vi "VeerAnemometers.vi"() -> ()   [LabVIEW 2011]
doc: "Use this VI with the UDP Sender VI. Run this VI first.\n\nThe UDP protocol differs from TCP in that there is no error-checking with the packets of information that are sent, and thus no guarantee whatsoever that an intended recipient will actually receive a given piece of data.\n\nUDP does offer the ability to \"broadcast\" data across a network--simply specify an IP Address of all ones (255.255.255.255) to attempt to broadcast information network-wide. Keep in mind that routers and other network hardware will generally refuse to forward the broadcast beyond certain points, so the extent of the broadcast will in practice be limited."
panel:
  out "Windspeed m/s 2":dbl(slide) scale=0.0..20.0
  out "Windspeed m/s":dbl(slide) scale=0.0..20.0
  out "Wind Direction":cluster{dbl, dbl}(knob) scale=0.0..360.0
  out "data out 3":string
  in  "Port 2":u16=61560
  out "data out":string
  in  "max bytes/read":i32=548
  in  "Port":u16=61559
  in  "stop":bool
  # "CPP Wind Engineering"
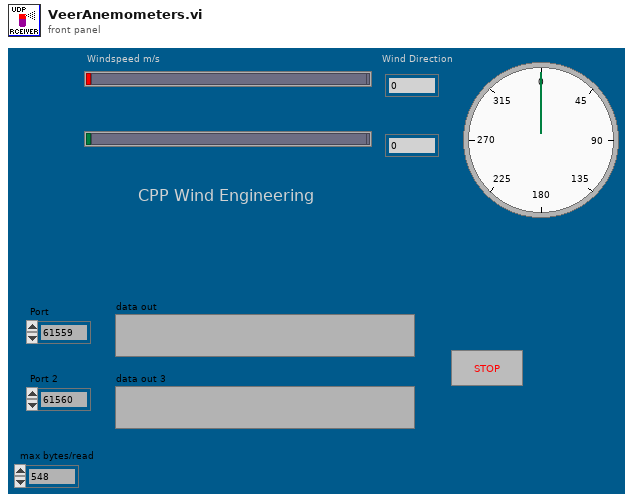
[diagram p1: front panel]
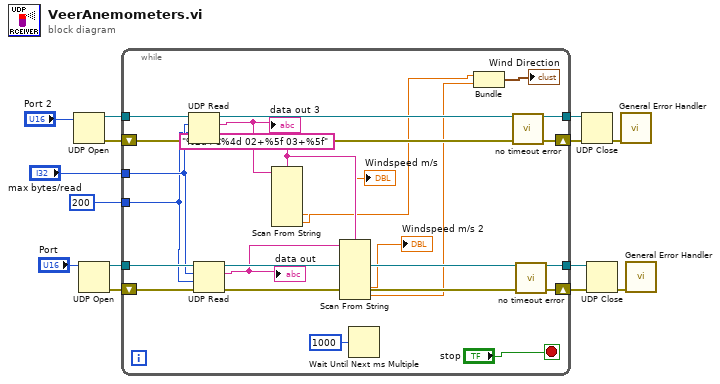
[diagram p0: block diagram]
diagram:
  n1 = UDP Open(11:"Port 2") -> (port=w3:refnum<k16>, 0:w2:errorcluster)  [unwired: 4 in, 1 out]
  n2 = UDP Open(11:"Port") -> (port=w12:refnum<k16>, 0:w13:errorcluster)  [unwired: 4 in, 1 out]
  n3 = while {
    tunnel: [w34] -> w11
    tunnel: w12 -> [w35]
    shift-left: w13 -> [w36]
    shift-right: [w32] -> w10
    tunnel: "max bytes/read" -> [w24]
    tunnel: 200 -> [w23]
    tunnel: [w27] -> w4
    tunnel: w3 -> [w26]
    shift-right: [w29] -> w5
    shift-left: w2 -> [w25]
    stop <- "stop" stop-if-true
    w19 = "%2d+C%4d 02+%5f 03+%5f" ("format string")
    n4 = UDP Read(connection ID=w26, max size (548)=w24, timeout ms (25000)=w23, 8:w25) -> (data out=w21:string, error out=w28:errorcluster, 3:w27:refnum<k16>)  [unwired: 2 out]
    "data out 3" <- w21
    n5 = UDP Read(connection ID=w35, max size (548)=w24, timeout ms (25000)=w23, 8:w36) -> (data out=w20:string, error out=w33:errorcluster, 3:w34:refnum<k16>)  [unwired: 2 out]
    "data out" <- w20
    n6 = Scan From String(format string=w19, input string=w21) -> (output 3=→"Windspeed m/s":dbl, output 4=w17:dbl)  [unwired: 8 in, 3 out]
    n7 = Scan From String(format string=w19, input string=w20) -> (output 3=→"Windspeed m/s 2":dbl, output 4=w18:dbl)  [unwired: 8 in, 3 out]
    n8 = Wait Until Next ms Multiple(millisecond multiple=u32 1000) -> ()  [unwired: 1 out]
    n9 = Bundle(w17, w18) -> (→"Wind Direction":cluster{dbl, dbl})  [unwired: 1 in]
    n10 = call "no timeout error.vi"("error in (no error)"=w28) -> ("error out"=w29:errorcluster)
    n11 = call "no timeout error.vi"("error in (no error)"=w33) -> ("error out"=w32:errorcluster)
  }
  n12 = UDP Close(connection ID=w4, 8:w5) -> (error out=w6:errorcluster)  [unwired: 1 out]
  n13 = UDP Close(connection ID=w11, 8:w10) -> (error out=w9:errorcluster)  [unwired: 1 out]
  n14 = call <vilib>:"General Error Handler.vi"("error in (no error)"=w6) -> ()  [unwired: 10 in, 5 out]
  n15 = call <vilib>:"General Error Handler.vi"("error in (no error)"=w9) -> ()  [unwired: 10 in, 5 out]
